vi "Interface.vi"(9 "EventsIn":T1, 10 "Events":T2) -> ()   [LabVIEW 2014, in "BuildSpecEditor.lvlib" / "InstallerSpecEditor.lvclass"]
uses:
  InstallerSpecEditor.lvclass
  GCMCore/Providers/Veritech_GCM/Support/Framework/_Plugins/_LVCMPlugin/GCMPlugin_EventsOut.ctl
  GCMCore/Providers/Veritech_GCM/Support/Framework/_Plugins/_LVCMPlugin/GCMPlugin_EventsIn.ctl
  <vilib>/AppBuilder/IB_RW_Project/IB_RW_Project_PropBag_Action.ctl
  GCMCore/Providers/Veritech_GCM/Support/Framework/_Plugins/GCMPlugin/GCMPlugin.lvclass
panel:
  in  "Version":cluster{"major":u16, "minor":u16, "update":u16}
  in  "AutoIncrement":bool caption="Auto-increment?"
  # "Warning: unchecking Auto-increment? doesn't work here. If you want to uncheck it, do it from native properties window."
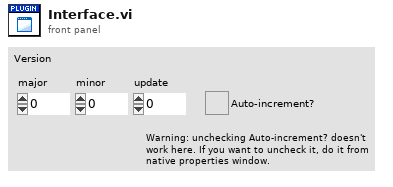
[diagram p1: front panel]
types:
  T1 = typedef "GCMPlugin.lvclass/GCMPlugin_EventsIn.ctl" = cluster{"Stop":refnum<user-event>, "ItemSelected":refnum<user-event>, "ItemDeselected":refnum<user-event>, "PluginActivated":refnum<user-event>, "PluginDeactivated":refnum<user-event>}
  T2 = typedef "GCMPlugin.lvclass/GCMPlugin_EventsOut.ctl" = cluster{"ItemEdited":refnum<user-event>}
  T3 = typedef "IB_RW_Project_PropBag_Action.ctl" = enum16{"read", "write", "clear", "readPrevious", "writePrevious", "clearPrevious"}
  T4 = cluster{"Item URL":string, "Item ID":string, "Item Index":i32, "Specific Type":string}
  T5 = typedef "ItemRef.ctl" = u64
  T6 = typedef "IB_RW_Project_Installer_Data.ctl" = cluster{"author":string, "productName":string, "buildSpecName":string, "hide":bool, "requireLVDevSys":bool, "autoIncrement":bool, "includeError":bool, "readmeID":string, "buildLocation":path, "mediaSize":u16, "language":T7, "productVersion":T8, "defaultDir":string, "web service itemIDs":string[]}
  T7 = typedef "CDK_sTypeDef_Languages.ctl" = u16
  T8 = typedef "CDK_sTypeDef_ProductVersion.ctl" = cluster{"Major":u8, "Minor":u8, "Update":u16}
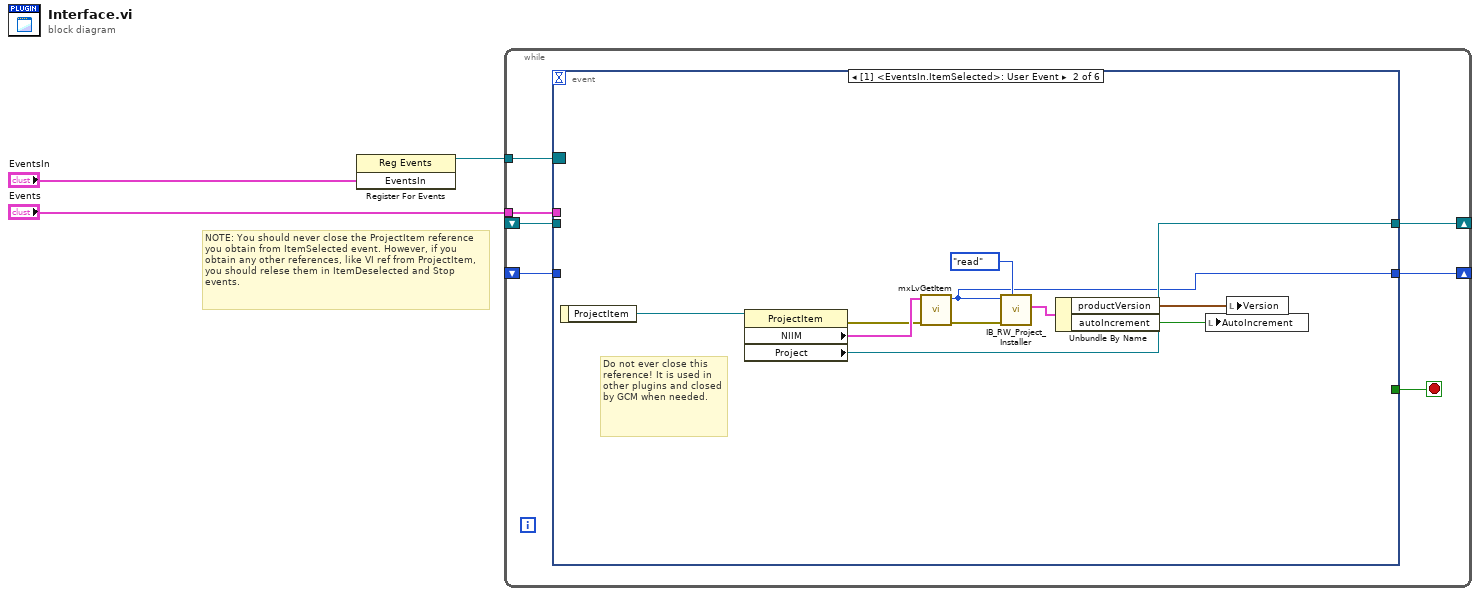
[diagram p0: block diagram]
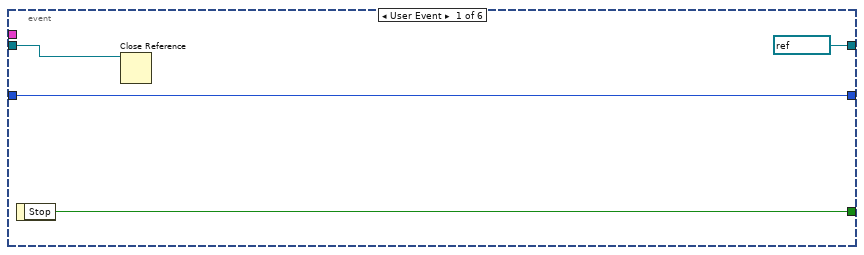
[diagram p2: hidden frame]
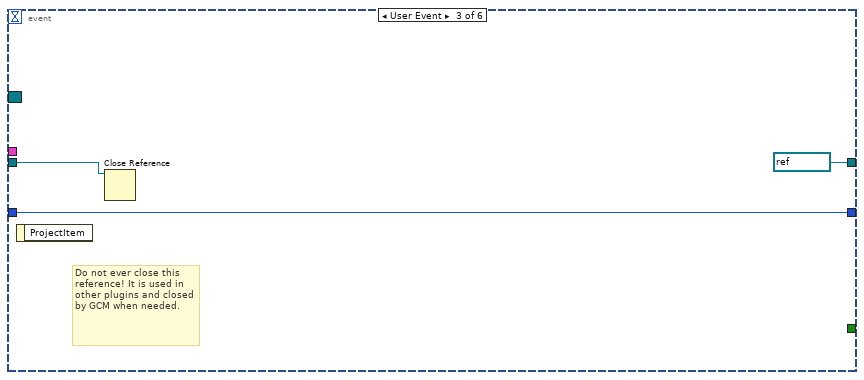
[diagram p3: hidden frame]
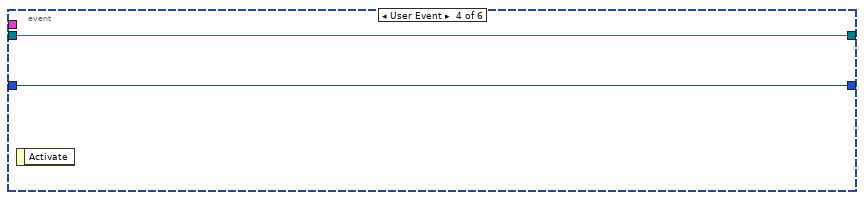
[diagram p4: hidden frame]
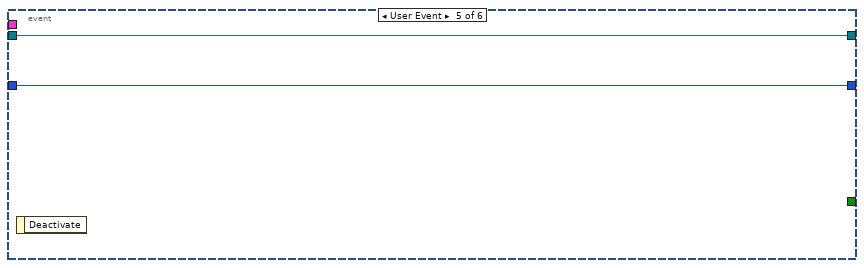
[diagram p5: hidden frame]
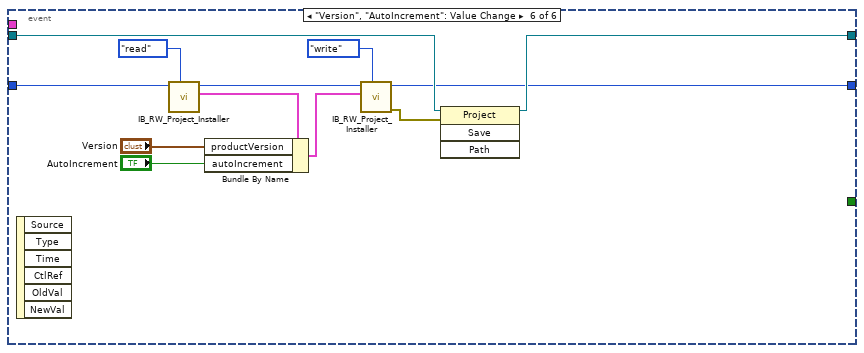
[diagram p6: hidden frame]
diagram:
  # "NOTE: You should never close the ProjectItem reference you obtain from ItemSelected event. However, if you obtain any other references, like VI ref from ProjectItem, you should relese them in ItemDeselected and Stop events."
  n1 = register-events("EventsIn") -> (reference out=w2:refnum<event-registration>)  [unwired: 2 in, 1 out]
  n2 = while {
    tunnel: w2 -> [w10]
    tunnel: "Events" -> [w9]
    shift-right: [w7] -> _
    shift-left: _ -> [w6]
    shift-right: [w5] -> _
    shift-left: _ -> [w4]
    stop <- w8 stop-if-true
    n3 = event shown="[1] <EventsIn.ItemSelected>: User Event" {
      selector: w10 -> [_ _ _ _ _ _]
      dyn-events: _ -> [_ _ _ _ _ _]
      timeout: _ -> [_ _ _ _ _ _]
      tunnel: w9 -> [_ _ _ _ _ _]
      tunnel: [w14 _ _ _ _ _] -> w8
      tunnel: [w13 w16 w27 w29 w31 w41] -> w7
      tunnel: w6 -> [w13 _ w27 w29 w31 w37]
      tunnel: [refnum<vi> refnum ("Project") w21 refnum<vi> refnum ("Project") w28 w30 w42] -> w5
      tunnel: w4 -> [w12 _ w26 w28 w30 w43]
      event User Event {
        n4 = event-data() -> ("Stop"=w14:bool)  [unwired: 1 in]
        n5 = Close Reference(reference=w12) -> ()  [unwired: 1 in, 1 out]
      }
      event User Event {
        # "Do not ever close this reference! It is used in other plugins and closed by GCM when needed."
        n6 = event-data() -> ("ProjectItem"=w24:refnum<vi>)  [unwired: 1 in]
        n7 = property class="ProjectItem"(reference=w24) -> (error out=w22:errorcluster, "NIIM"=w23:T4, "Project"=w21:refnum<vi>)  [unwired: 1 in, 1 out]
        n8 = call <resource>:"mxLvGetItem.vi"("error in"=w22, "NIIM"=w23) -> ("error out"=w19:errorcluster, "Item"=w16:T5)  [unwired: 8 in]
        n9 = call <vilib>:"IB_RW_Project_Installer.vi"("action"=IB_RW_Project_PropBag_Action."read", "error in (no error)"=w19, "Object In"=w16) -> ("Installer out"=w18:T6)  [unwired: 6 in, 2 out]
        n10 = Unbundle By Name(w18) -> ("productVersion"=w17:T8, "autoIncrement"=w15:bool)
        n11 = local write "AutoIncrement"(w15) -> ()
        n12 = local write "Version"(w17) -> ()
      }
      event User Event {
        # "Do not ever close this reference! It is used in other plugins and closed by GCM when needed."
        n13 = event-data() -> ()  [unwired: 1 in, 1 out]
        n14 = Close Reference(reference=w26) -> ()  [unwired: 1 in, 1 out]
      }
      event User Event {
        n15 = event-data() -> ()  [unwired: 1 in, 1 out]
      }
      event User Event {
        n16 = event-data() -> ()  [unwired: 1 in, 1 out]
      }
      event "Version", "AutoIncrement": Value Change {
        n17 = event-data() -> ()  [unwired: 1 in, 6 out]
        n18 = call <vilib>:"IB_RW_Project_Installer.vi"("action"=IB_RW_Project_PropBag_Action."read", "Object In"=w37) -> ("Installer out"=w35:T6, "Object Out"=w36:T5)  [unwired: 7 in, 1 out]
        n19 = Bundle By Name(cluster=w35, "productVersion"="Version", "autoIncrement"="AutoIncrement") -> (w34:T6)
        n20 = call <vilib>:"IB_RW_Project_Installer.vi"("action"=IB_RW_Project_PropBag_Action."write", "Installer in"=w34, "Object In"=w36) -> ("error out"=w39:errorcluster, "Object Out"=w41:T5)  [unwired: 6 in, 1 out]
        n21 = invoke class="Project" method="Save"(reference=w43, error in=w39) -> (reference out=w42:refnum<vi>)  [unwired: 2 in, 3 out]
      }
    }
  }
